vi "AddQualisysData.vi"(4 "QualisysDataType":enum16{"6DOF", "3DTracking"}(ring), 5 "sortie d'erreur":errorcluster caption="entrée d'erreur", 6 "FichierQualisys":path, 7 "FichierTDMS":path, 8 "NomProjectIN":string) -> (0 "error out":errorcluster, 1 "QualisysMergeInfo":string, 2 "MergedFile":path, 3 "NomProjectOUT":string)   [LabVIEW 2015]
uses:
  DefDeType/WhichPath.ctl
  <vilib>/Waveform/WDTOps.llb/WDT Waveform Duration DBL.vi
  <vilib>/Waveform/WDTOps.llb/WDT Get Waveform Subset DBL.vi
panel:
  out "dt":dbl
  out "Tableau":dbl[](array[numeric])
  out "DurationDifference":dbl
  out "NbVoiesTDMS":i32
  out "NbVoiesQualisys":i32
  out "NbVoiesFinal":i32
  out "MergedWaveForms":waveform(dbl)[](graph)
  out "TDMSDuree":dbl caption="TDMSduree" format="%0.2f"
  out "QualisysDuree":dbl format="%0.2f"
  out "TimeStampDiff(sec)":dbl
  out "QualisysMergeMessage":string
  out "TDMSTimeStamp":timestamp
  out "TDMSdt":dbl
  out "QualisysTimeStamp":timestamp
  out "Qualisysdt":dbl
  out "TDMSWaveForms":waveform(dbl)[](graph)
  out "QualisysWaveforms":waveform(dbl)[](graph)
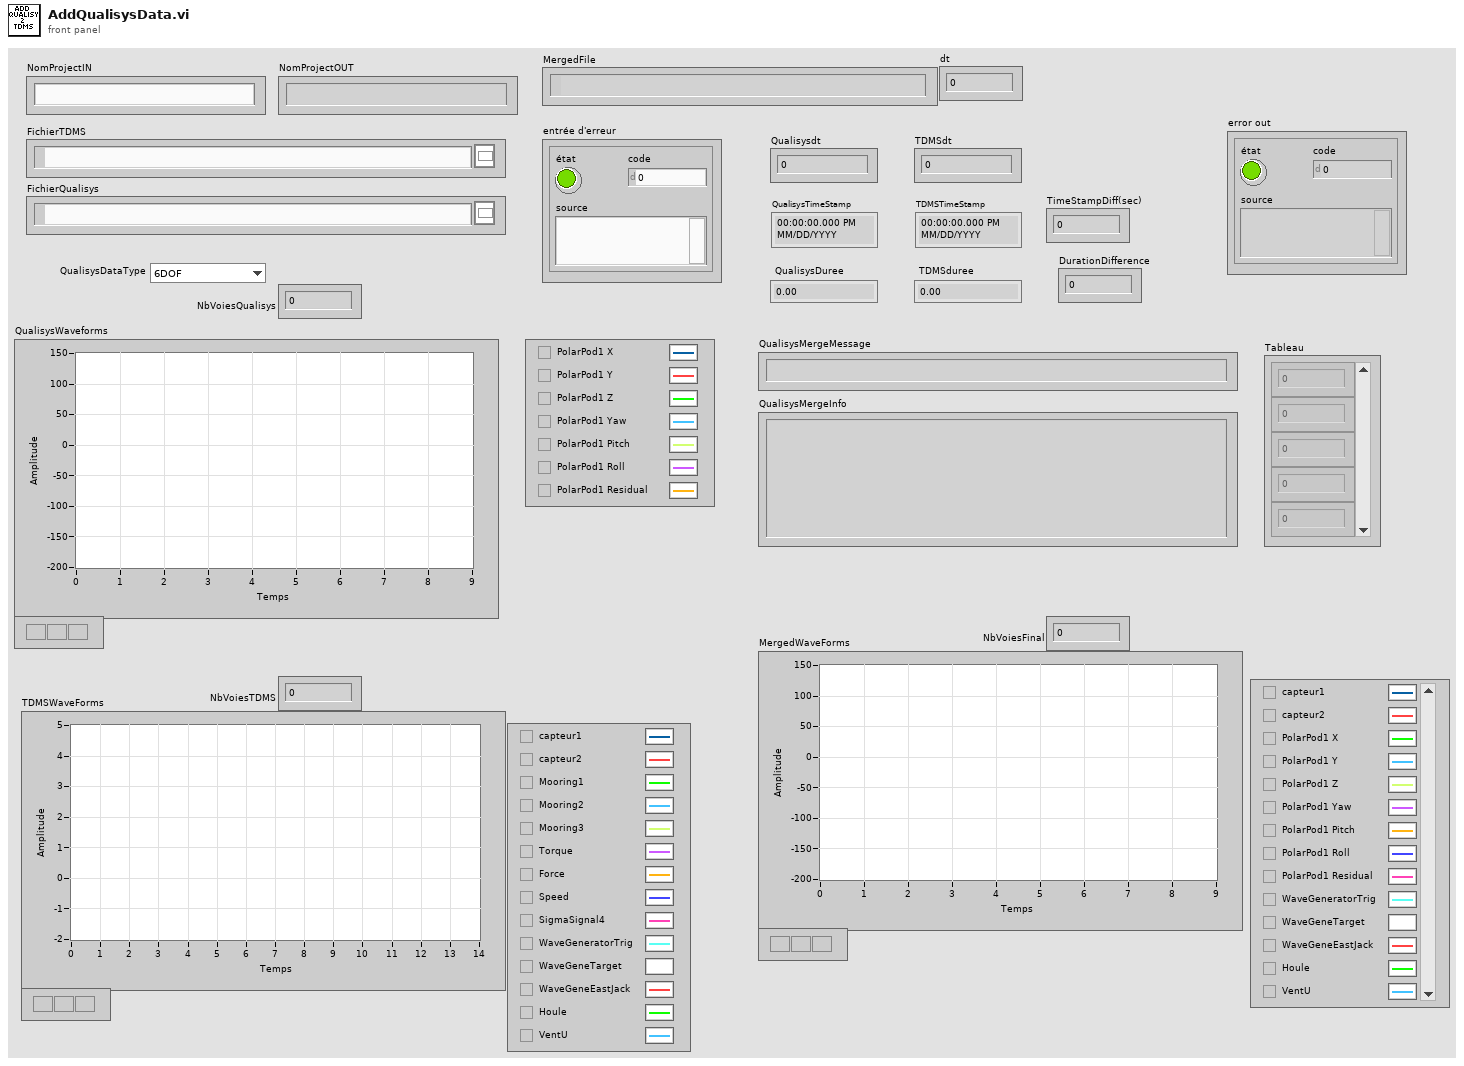
[diagram p1: front panel]
types:
  T1 = enum16{"open", "open or create", "create or replace", "create", "open (read-only)"}
  T2 = typedef "WhichPath.ctl" = enum16{"DossierProjet", "Config", "Meas", "MeasSuitCase", "MeasOnBoard", "MeasQualisys", "MeasTDMS", "MeasHexapode", "MeasNortek", "Fig", "Res"}
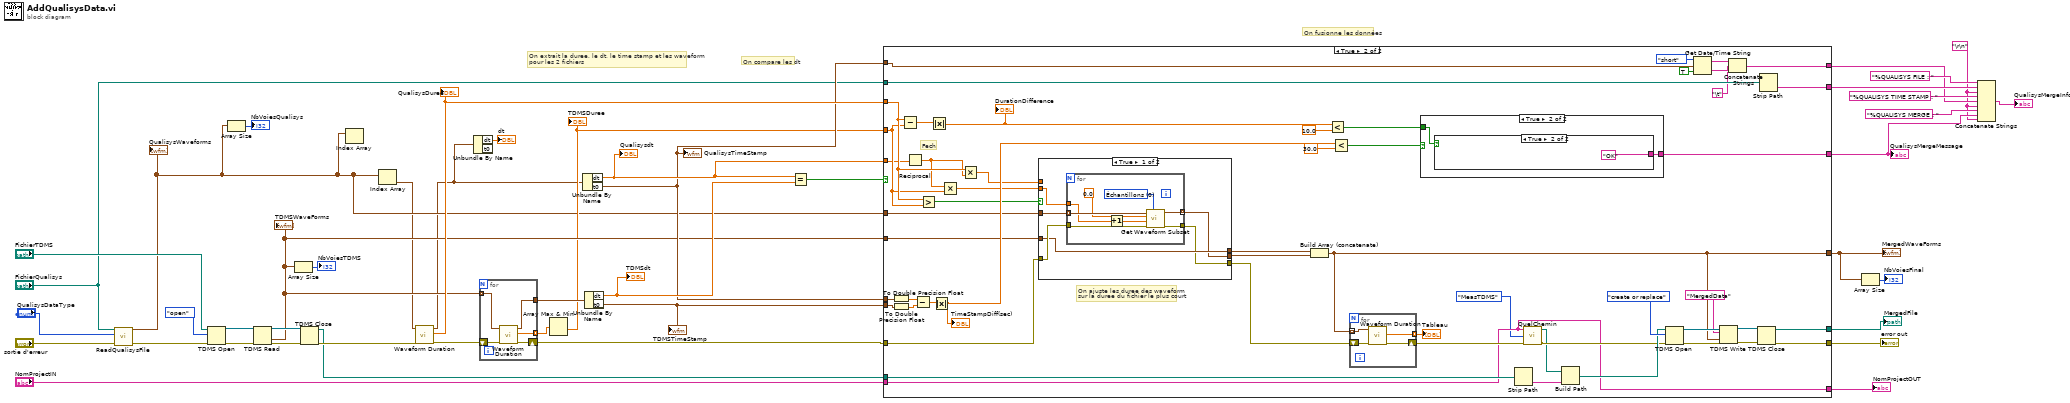
[diagram p0: block diagram]
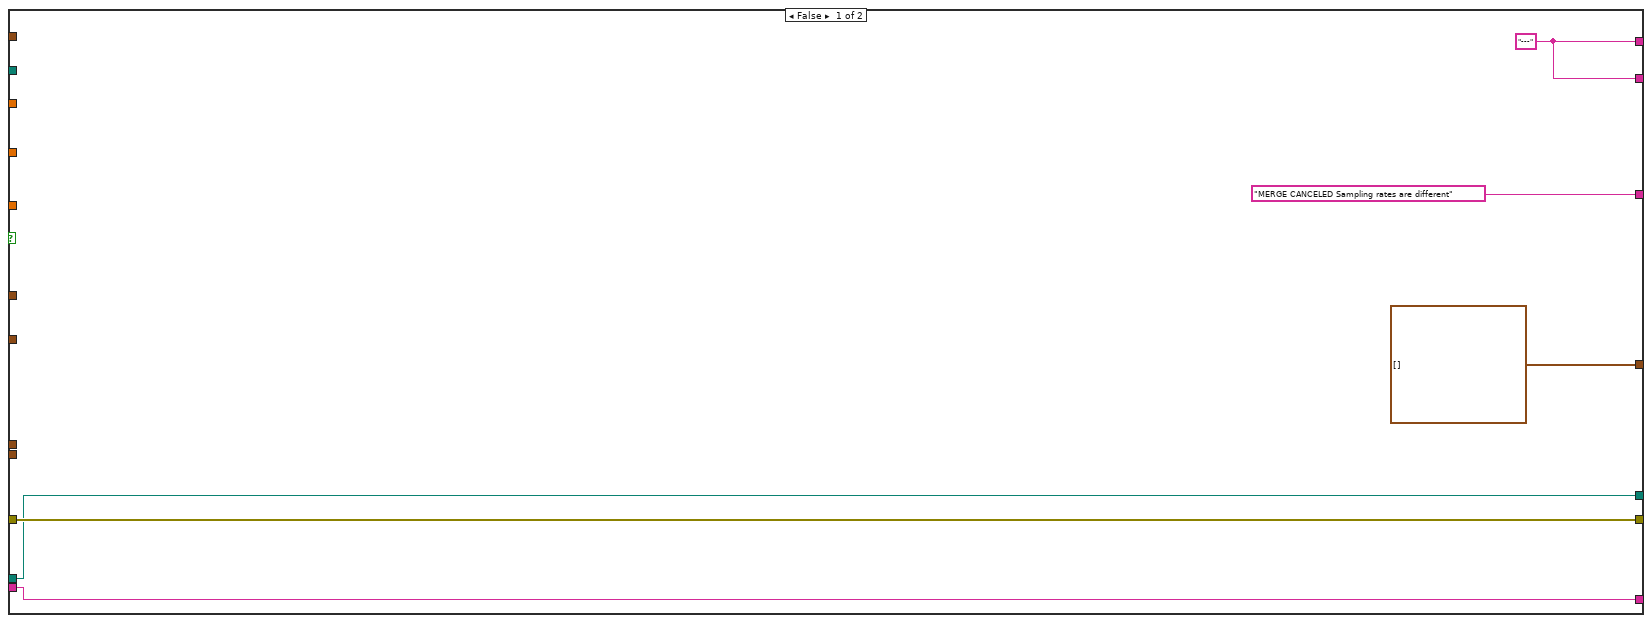
[diagram p2: hidden frame]
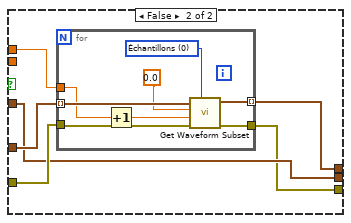
[diagram p3: hidden frame]
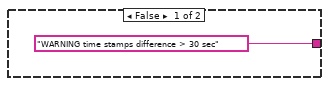
[diagram p4: hidden frame]
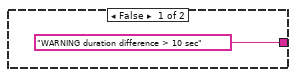
[diagram p5: hidden frame]
diagram:
  w16 = "\r\n"
  # "On fusionne les données"
  # "On compare les dt"
  # "On extrait la duree, le dt, le time stamp et les waveform\npour les 2 fichiers"
  n1 = call "ReadQualisysFile.vi"("sortie d'erreur"="sortie d'erreur", "QualisysDataType"="QualisysDataType", "FichierQualisys"="FichierQualisys") -> ("error out"=w7:errorcluster, "QualisysWaveforms"=w5:waveform(dbl)[])  [unwired: 3 in]
  "QualisysWaveforms" <- w5
  n2 = TDMS Open(8:w7, 10:T1."open" ("opération (0 : open)"), 11:"FichierTDMS") -> (0:w42:errorcluster, 3:w41:refnum<k34>)  [unwired: 4 in]
  n3 = Array Size(array=w5) -> (size(s)=→"NbVoiesQualisys":i32)
  n4 = TDMS Read(0:w41, 11:w42) -> (4:w39:refnum<k34>, 10:w11:waveform(dbl)[], 15:w40:errorcluster)  [unwired: 6 in, 3 out]
  "TDMSWaveForms" <- w11
  n5 = Array Size(array=w11) -> (size(s)=→"NbVoiesTDMS":i32)
  n6 = TDMS Close(8:w40, 11:w39) -> (0:w34:errorcluster, 3:w24:path)
  n7 = Index Array(array=w5) -> ()  [unwired: 1 in, 1 out]
  n8 = Index Array(array=w5) -> (element=w3:waveform(dbl))  [unwired: 1 in]
  n9 = call-poly <vilib>:"Waveform Duration.vi"("error in (no error)"=w34, "waveform in"=w3) -> ("error out"=w35:errorcluster, "duration"=w26:dbl, "waveform out"=w2:waveform(dbl))  [unwired: 7 in]
  "QualisysDuree" <- w26
  n10 = Unbundle By Name(w2) -> ("dt"=→"dt":dbl)  [unwired: 1 out]
  n11 = for {
    tunnel: [w47] -> w32
    tunnel: [w46] -> w10 mode=indexing
    shift-right: [w48] -> w33
    shift-left: w35 -> [w49]
    tunnel: w11 -> [w45] mode=indexing
    n12 = call-poly <vilib>:"Waveform Duration.vi"("error in (no error)"=w49, "waveform in"=w45) -> ("error out"=w48:errorcluster, "duration"=w46:dbl, "waveform out"=w47:waveform(dbl))  [unwired: 7 in]
  }
  n13 = Array Max & Min(array=w10) -> (min value=w9:dbl)  [unwired: 3 out]
  "TDMSDuree" <- w9
  n14 = Unbundle By Name(w2) -> ("dt"=w25:dbl, "t0"=w20:timestamp)
  "Qualisysdt" <- w25
  "QualisysTimeStamp" <- w20
  n15 = Unbundle By Name(w32) -> ("dt"=w38:dbl, "t0"=w36:timestamp)
  "TDMSdt" <- w38
  "TDMSTimeStamp" <- w36
  n16 = Equal?(x=w25, y=w38) -> (x = y?=w37:bool)
  n17 = case shown="True" w37 {
    tunnel: w33 -> [w53 w91]
    tunnel: ["MERGE CANCELED Sampling rates are different" ("QualisysMergeMessage") w101] -> w17
    tunnel: w20 -> [_ w108]
    tunnel: w36 -> [_ w106]
    tunnel: w11 -> [_ w92]
    tunnel: w5 -> [_ w93]
    tunnel: [waveform(dbl)[] [] w75] -> w31
    tunnel: [w53 w80] -> w27
    tunnel: w26 -> [_ w89]
    tunnel: w9 -> [_ w88]
    tunnel: w25 -> [_ w85]
    tunnel: w24 -> [w51 w63]
    tunnel: "FichierQualisys" -> [_ w73]
    tunnel: [w52 w72] -> w21
    tunnel: w20 -> [_ w71]
    tunnel: [w52 w65] -> w19
    tunnel: [w51 w64] -> w14
    tunnel: "NomProjectIN" -> [w50 w57]
    tunnel: [w50 w57] -> w12
    frame False {
      w52 = "---"
    }
    frame True {
      # "On ajuste les duree des waveform \nsur la duree du fichier le plus court"
      # "Fech"
      n18 = To Double Precision Float(number=w108) -> (double precision float=w107:dbl)
      n19 = To Double Precision Float(number=w106) -> (double precision float=w105:dbl)
      n20 = Subtract(x=w89, y=w88) -> (x-y=w95:dbl)
      n21 = Reciprocal(x=w85) -> (1/x=w82:dbl)
      n22 = Subtract(x=w107, y=w105) -> (x-y=w104:dbl)
      n23 = Greater?(x=w89, y=w88) -> (0:w94:bool)
      n24 = Absolute Value(x=w95) -> (abs(x)=w98:dbl)
      "DurationDifference" <- w98
      n25 = Absolute Value(x=w104) -> (abs(x)=w103:dbl)
      "TimeStampDiff(sec)" <- w103
      n26 = Multiply(x=w82, y=w88) -> (x*y=w83:dbl)
      n27 = Multiply(x=w89, y=w82) -> (x*y=w84:dbl)
      n28 = case shown="True" w94 {
        tunnel: w93 -> [w114 w125]
        tunnel: w92 -> [w112 w127]
        tunnel: w84 -> [_ w123]
        tunnel: w83 -> [w111 _]
        tunnel: w91 -> [w113 w128]
        tunnel: [w109 w124] -> w90
        tunnel: [w112 w126] -> w87
        tunnel: [w110 w125] -> w86
        frame True {
          n29 = for {
            tunnel: w114 -> [w122] mode=indexing
            tunnel: w113 -> [w121]
            tunnel: [w120] -> w109
            tunnel: w111 -> [w118]
            tunnel: [w117] -> w110 mode=indexing
            w116 = u16 0 items=["Échantillons", "Temps relatif"] ("start/duration format")
            n30 = Increment(x=w118) -> (x+1=w115:dbl)
            n31 = call-poly <vilib>:"Get Waveform Subset.vi"("start/duration format"=w116, "error in (no error)"=w121, "duration"=w115, "start samples/time"=0.0, "waveform in"=w122) -> ("error out"=w120:errorcluster, "waveform out"=w117:waveform(dbl))  [unwired: 1 in, 2 out]
          }
        }
        frame False {
          n32 = for {
            tunnel: w127 -> [w136] mode=indexing
            tunnel: w128 -> [w135]
            tunnel: [w134] -> w124
            tunnel: w123 -> [w132]
            tunnel: [w131] -> w126 mode=indexing
            w130 = u16 0 items=["Échantillons", "Temps relatif"] ("start/duration format")
            n33 = Increment(x=w132) -> (x+1=w129:dbl)
            n34 = call-poly <vilib>:"Get Waveform Subset.vi"("start/duration format"=w130, "error in (no error)"=w135, "duration"=w129, "start samples/time"=0.0, "waveform in"=w136) -> ("error out"=w134:errorcluster, "waveform out"=w131:waveform(dbl))  [unwired: 1 in, 2 out]
          }
        }
      }
      n35 = Build Array (concatenate)(w87, w86) -> (w75:waveform(dbl)[])
      n36 = Less?(x=w98, y=10.0) -> (x < y?=w97:bool)
      n37 = Less?(x=w103, y=30.0) -> (x < y?=w100:bool)
      n38 = for {
        shift-right: [w139] -> w60
        shift-left: w90 -> [w140]
        tunnel: w75 -> [w138] mode=indexing
        tunnel: [w137] -> w96 mode=indexing
        n39 = call-poly <vilib>:"Waveform Duration.vi"("error in (no error)"=w140, "waveform in"=w138) -> ("error out"=w139:errorcluster, "duration"=w137:dbl)  [unwired: 7 in, 1 out]
      }
      "Tableau" <- w96
      n40 = case shown="True" w100 {
        tunnel: ["WARNING time stamps difference > 30 sec" ("QualisysMergeMessage") w143] -> w101
        tunnel: w97 -> [_ w142]
        frame False {
        }
        frame True {
          n41 = case shown="True" w142 {
            tunnel: ["WARNING duration difference > 10 sec" ("QualisysMergeMessage") "OK" ("QualisysMergeMessage")] -> w143
            frame False {
            }
            frame True {
            }
          }
        }
      }
      n42 = Strip Path(path=w63) -> (name=w62:string)  [unwired: 1 out]
      n43 = call "QuelChemin.vi"("Entrée d'erreur"=w60, "WhichPath?"=WhichPath."MeasTDMS", "NomProjet"=w57) -> ("Sortie d'erreur"=w59:errorcluster, "SurDisqueLocal"=w58:path)  [unwired: 1 out]
      n44 = Build Path(base path=w58, name or relative path=w62) -> (appended path=w61:path)
      n45 = TDMS Open(8:w59, 10:T1."create or replace" ("opération (0 : open)"), 11:w61) -> (0:w79:errorcluster, 3:w77:refnum<k34>)  [unwired: 4 in]
      n46 = Get Date/Time String(date format (0)=enum16{"short", "long", "abbreviated"}."short" ("format de date (0)"), seconds (now)=w71, want seconds? (F)=TRUE ("secondes ? (F)")) -> (date string=w68:string, time string=w67:string)
      n47 = TDMS Write(0:w77, 5:"MergedData" ("nom du groupe en entrée (Sans titre)"), 9:w75, 11:w79) -> (4:w76:refnum<k34>, 15:w78:errorcluster)  [unwired: 2 in, 2 out]
      n48 = Concatenate Strings(w68, "\t", w67) -> (w65:string)
      n49 = TDMS Close(8:w78, 11:w76) -> (0:w80:errorcluster, 3:w64:path)
      n50 = Strip Path(path=w73) -> (name=w72:string)  [unwired: 1 out]
    }
  }
  "QualisysMergeMessage" <- w17
  "MergedWaveForms" <- w31
  "error out" <- w27
  "MergedFile" <- w14
  "NomProjectOUT" <- w12
  n51 = Array Size(array=w31) -> (size(s)=→"NbVoiesFinal":i32)
  n52 = Concatenate Strings("%QUALISYS FILE : " ("chaîne"), w21, w16, "%QUALISYS TIME STAMP : " ("chaîne"), w19, w16, "%QUALISYS MERGE : " ("chaîne"), w17, w16) -> (→"QualisysMergeInfo":string)
